vi "MainScreen.vi"() -> ()   [LabVIEW 2020]
uses:
  Source/PN.ctl
  Source/NewPNConfig.ctl
  Source/InputPlanning.ctl
  <vilib>/Utility/miscctls.llb/LVRowAndColumnTypeDef.ctl
  85a98836-3ca8-4481-b4b7-f46a48c72065.vi
  <vilib>/Array/Sort 2D Array - Pop Stack.vi
  <vilib>/Array/Sort 2D Array - Push Stack.vi
  <vilib>/Utility/config.llb/Read Key (String).vi
  <vilib>/Utility/config.llb/Write Key (String).vi
  <vilib>/Utility/file.llb/Read Delimited Spreadsheet (string).vi
  <vilib>/Utility/file.llb/Write Delimited Spreadsheet (string).vi
  <vilib>/regexp/Match Regular Expression.xnode
  <vilib>/Utility/config.llb/NI_LVConfig.lvlib
panel:
  out "error out 4":errorcluster
  out "Version":string
  out "Boolean":bool
  out "ConfigPath":string
  out "Check":dbl
  out "TempFolder":string
  out "SeqPath":string
  in  "stop":bool
  out "TestStandPath":string
  in  "Tab1":T1(tab)
  in  "CurrentStatus":string[][](table)
  in  "Remove Button":bool
  out "CurrentQueue":string[][](table)
  in  "SAVE_Plan":bool
  in  "RESET_Queue":bool
  in  "InputParameter":T2
  in  "EditFlow":bool
  in  "SAVEConfig":bool
  in  "ConfigLoad":T3 {"Screw 8" items=["0", "1", "2", "3", "4", "5", "6", "7", "8", "9", "10"]; "Screw 7" items=["0", "1", "2", "3", "4", "5", "6", "7", "8", "9", "10"]; "Screw 6" items=["0", "1", "2", "3", "4", "5", "6", "7", "8", "9", "10"]; "Screw 5" items=["0", "1", "2", "3", "4", "5", "6", "7", "8", "9", "10"]; "Screw 4" items=["0", "1", "2", "3", "4", "5", "6", "7", "8", "9", "10"]; "Screw 3" items=["0", "1", "2", "3", "4", "5", "6", "7", "8", "9", "10"]; "Screw 2" items=["0", "1", "2", "3", "4", "5", "6", "7", "8", "9", "10"]; "M6_Camera" items=["0", "1", "2", "3", "4", "5", "6", "7", "8", "9", "10", "11", "12", "13", "14", "15", "16", "17", "18", "19", "20", "21", "22", "23", "24", "25", "26", "27", "28", "29", "30"]; "L/R" items=["NA", "RHD-VAC", "RHD-HVAC", "LHD-VAC", "LHD-HVAC"]}
  out "Layout":string[](array[string])=["VALEO PN", "LEFT/RIGHT", "SCREW"]
  in  "CurrentSeq":T4
  in  "String 2":string="EDIT PN"
  in  "CreateNewPN":bool
  in  "String":string="NEW PN"
  in  "New PN":string
  in  "Note":string[](array[string])
  in  "Control":bool[][](array[boolean])
  out "Input":bool[][](array[boolean])
  out "MAP":string[][](array[string])
  out "Slave Status":u32[](array[colorbox])
  in  "ManualMachine":bool
  in  "Select PN to send to Machine":T4
  in  "Select Machine for Manual Test":T4
  in  "StartRun":bool
  # "s1"
  # "s2"
  # "s3"
  # "s4"
  # "s5"
  # "s6"
  # "s7"
  # "s8"
  # "s9"
  # "s10"
  # "s11"
  # "s12"
  # "s13"
  # "s14"
  # "s15"
  # "s16"
  # "s17"
  # "s18"
  # "s19"
  # "s20"
  # "s21"
  # "s22"
  # "s23"
  # "s24"
  # "s25"
  # "s26"
  # "s27"
  # "s28"
  # "s29"
  # "s30"
  # "s31"
  # "P2"
  # "P1"
  # "P3"
  # "P0"
  # "P0"
  # "P1"
  # "P2"
  # "P3"
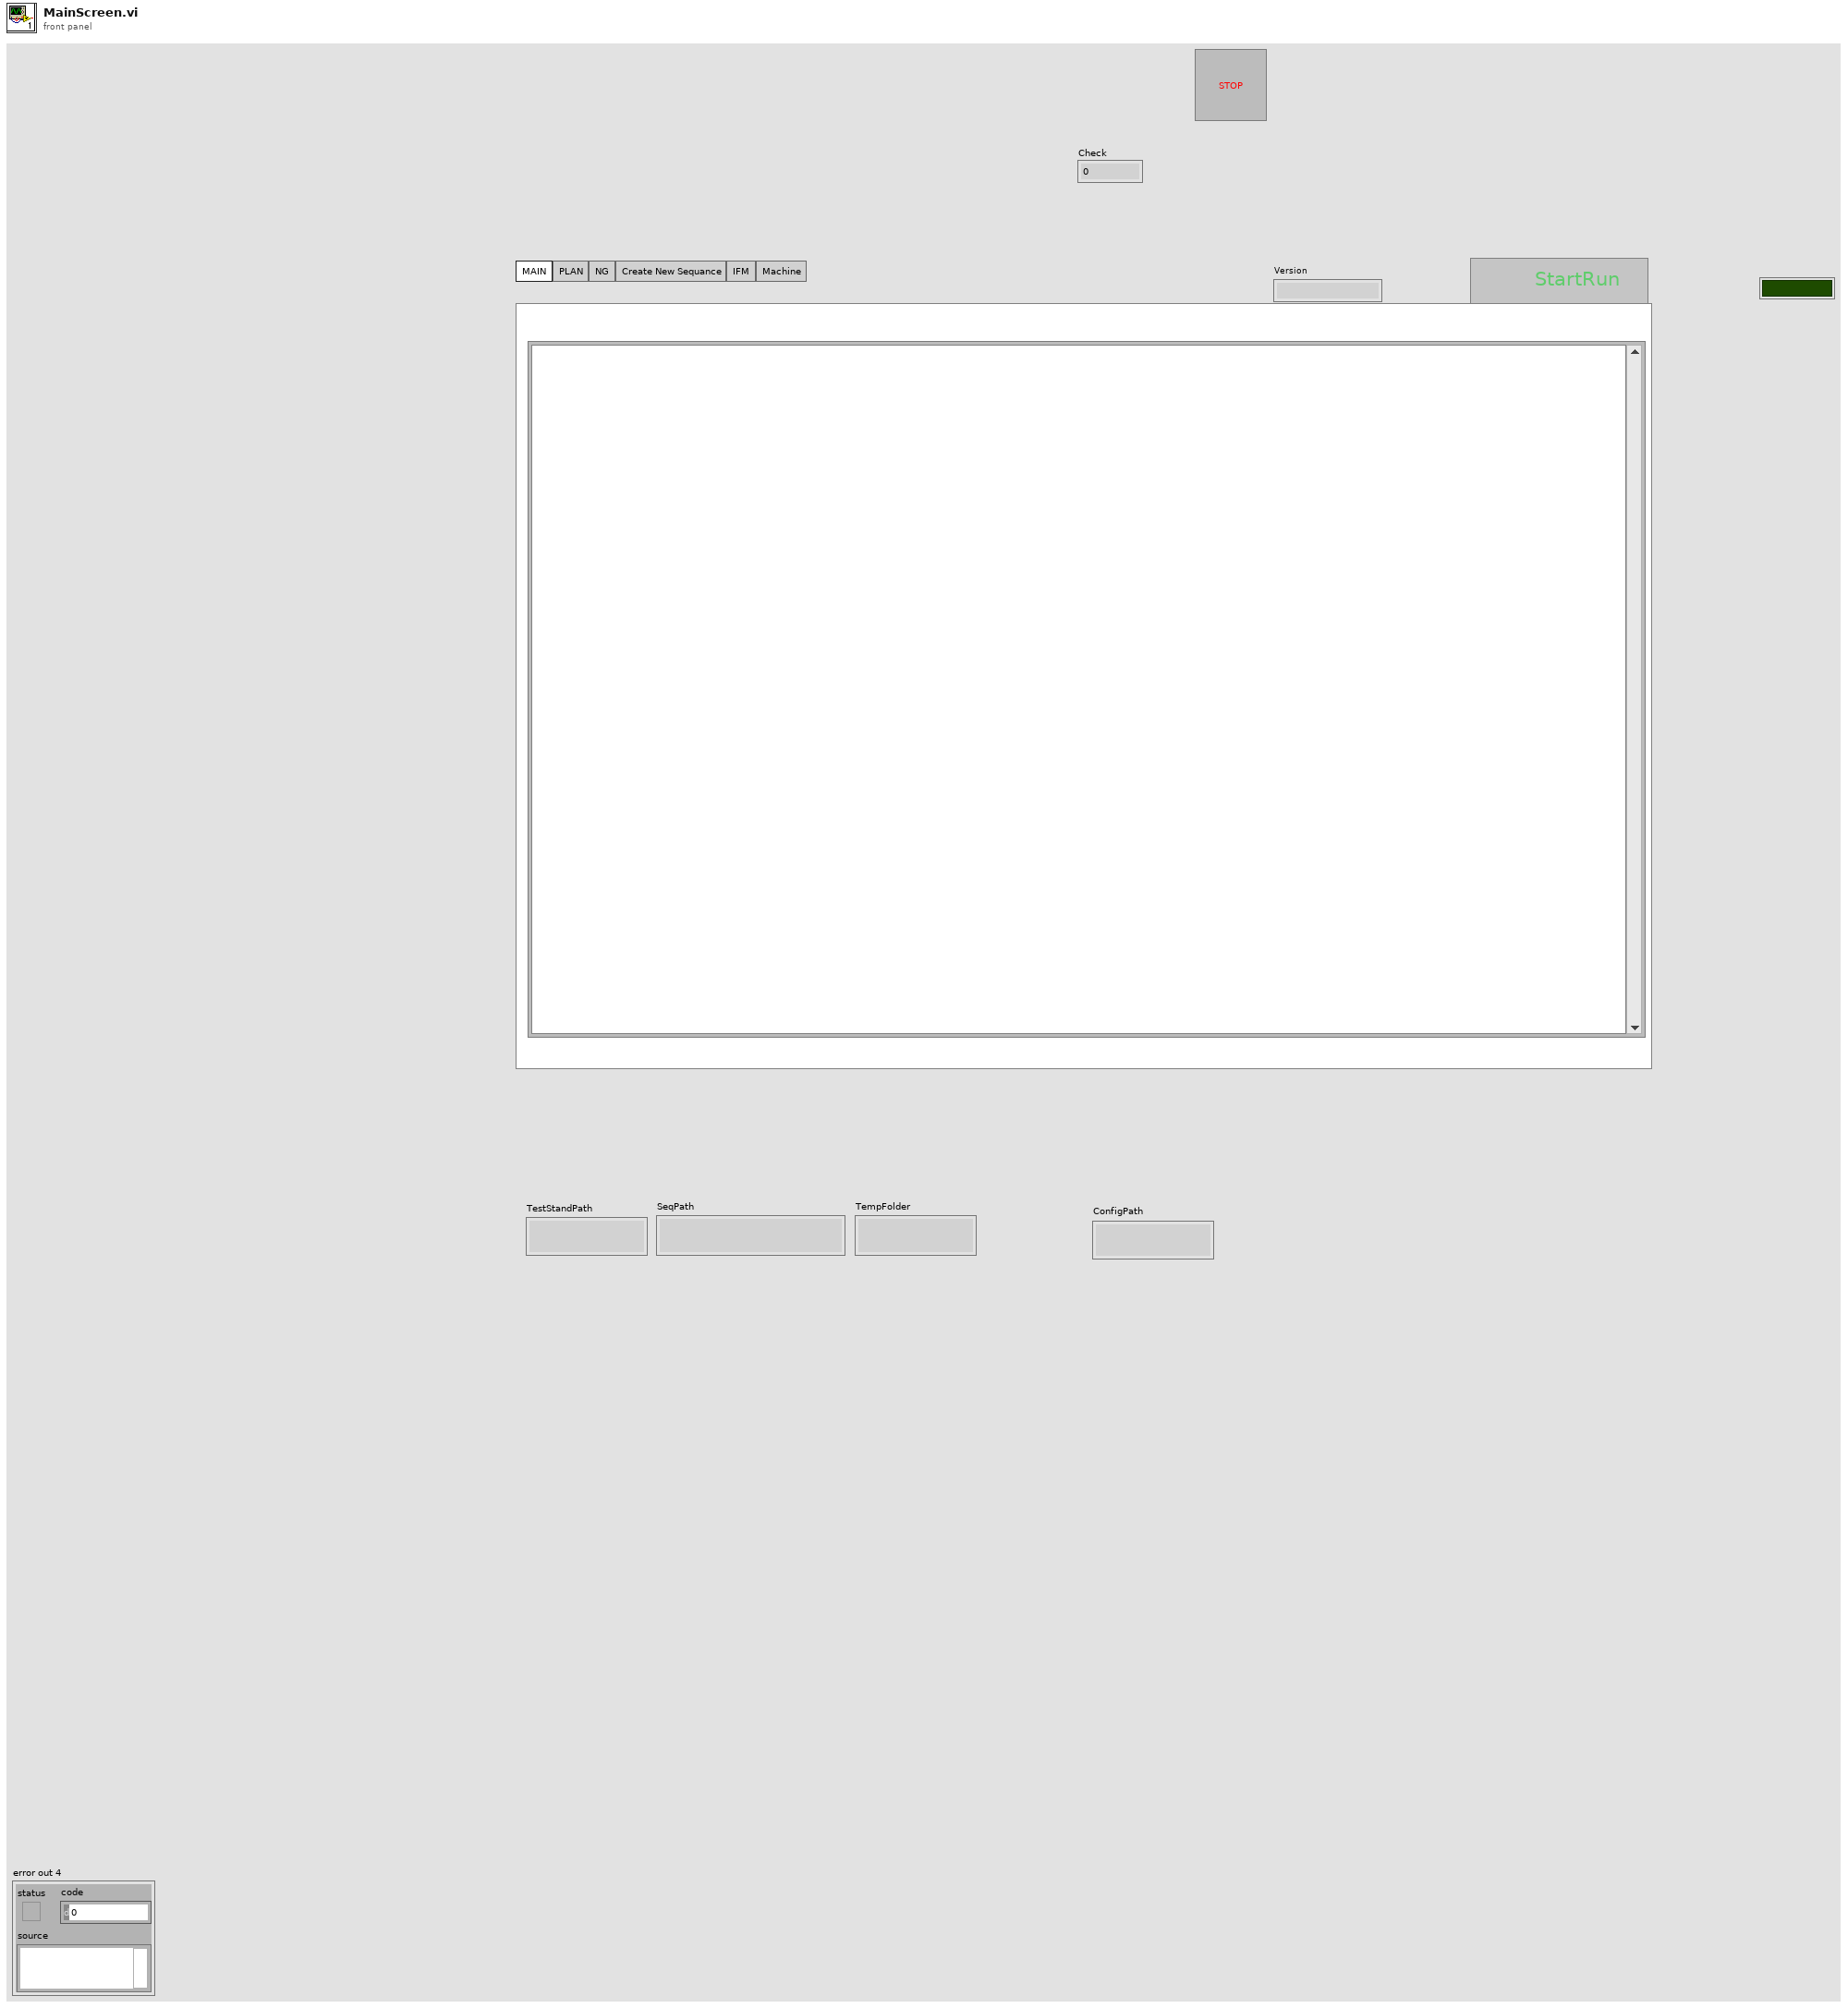
[diagram p1: front panel]
types:
  T1 = enum32{"MAIN", "PLAN", "NG", "Create New Sequance", "IFM", "Machine"}
  T2 = typedef "InputPlanning.ctl" = cluster{"Count":i16, "PN":string}[]
  T3 = typedef "NewPNConfig.ctl" = cluster{"L/R":u8, "PN":string, "M6_Camera":u16, "Screw 2":u16, "Screw 3":u16, "Screw 4":u16, "Screw 5":u16, "Screw 6":u16, "Screw 7":u16, "Screw 8":u16}
  T4 = typedef "PN.ctl" = string
  T5 = enum8{"Enabled", "Disabled", "Disabled and Grayed Out"}
  T6 = enum32{"MAIN", "PLAN", "NG", "Create New Sequance"}
  T7 = typedef "NI_LVConfig.lvlib/Config Data RefNum.ctl" = refnum<k1>
  T8 = typedef "LVRowAndColumnTypeDef.ctl" = cluster{"Row":i32, "Column":i32}
  T9 = cluster{"FileVersion":string, "FileMajorPart":i32, "FileMinorPart":i32, "FileBuildPart":i32, "FilePrivatePart":i32, "Language":string, "LegalCopyright":string, "FileDescription":string, "CompanyName":string, "ProductName":string, "InternalName":string}
  T10 = cluster{"Read Access":enum8{"Allowed", "Required", "None"}, "Write Access":enum8{"Allowed", "Required", "None"}}
  T11 = enum16{"open", "replace", "create", "open or create", "replace or create", "replace or create with confirmation"}
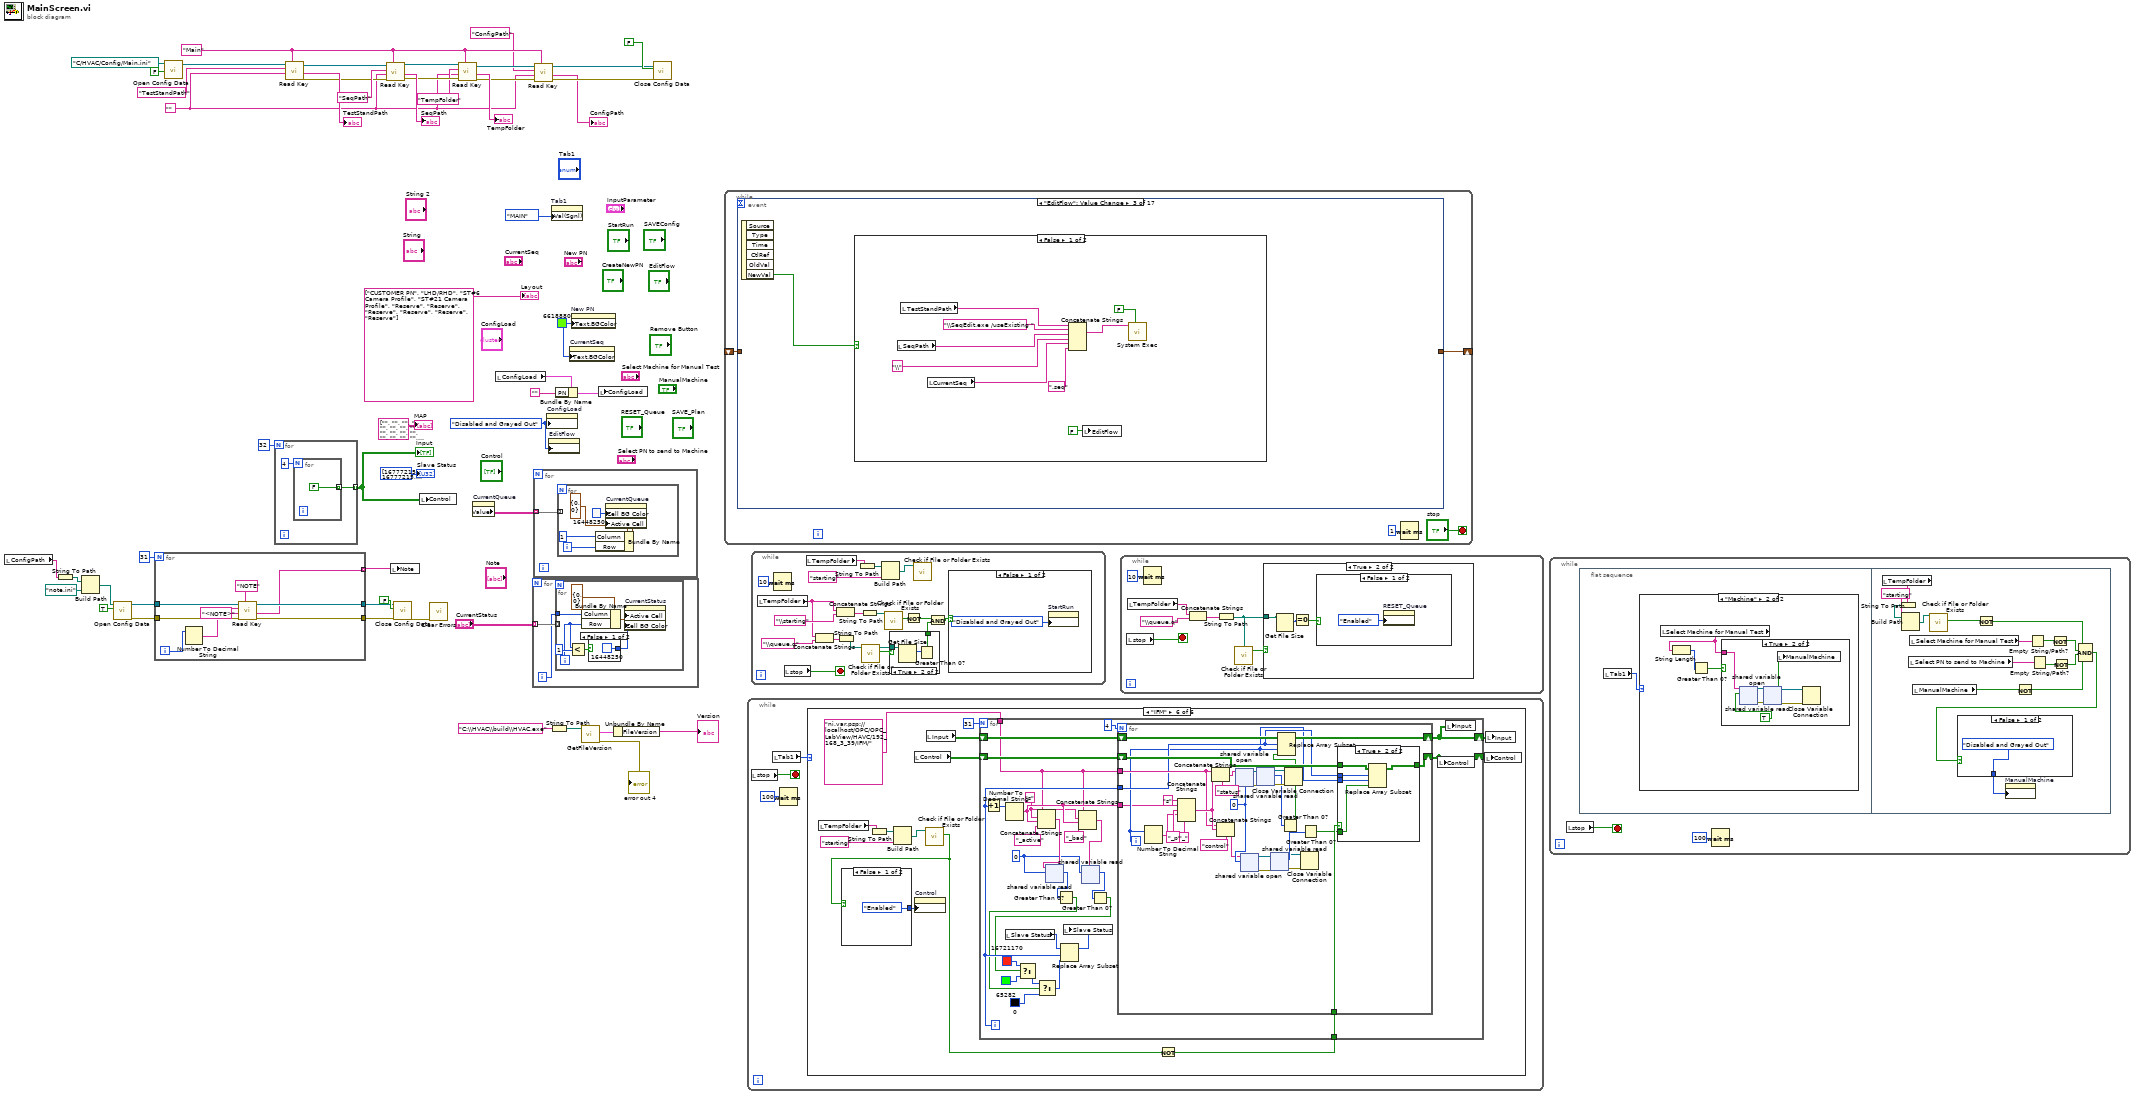
[diagram p0: block diagram]
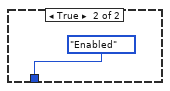
[diagram p4: hidden frame]
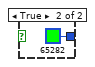
[diagram p5: hidden frame]
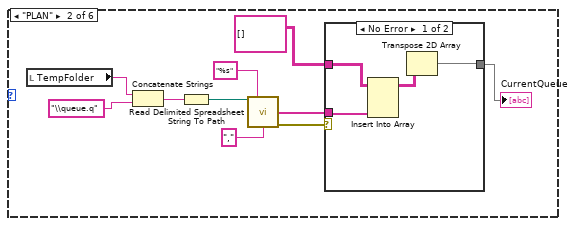
[diagram p7: hidden frame]
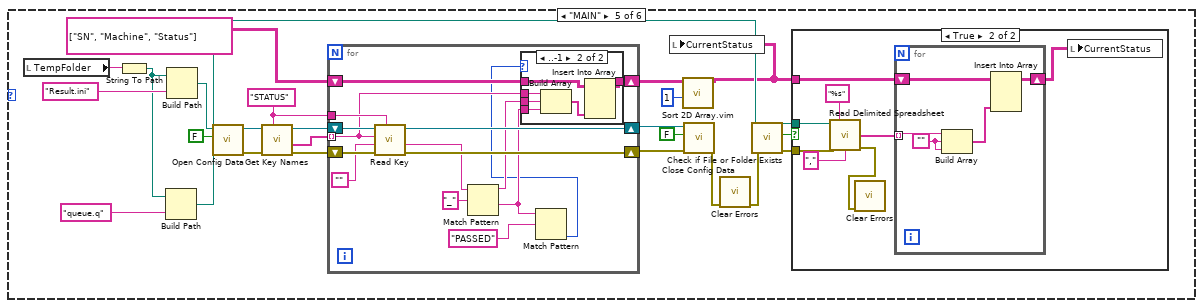
[diagram p11: hidden frame]
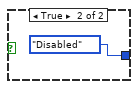
[diagram p14: hidden frame]
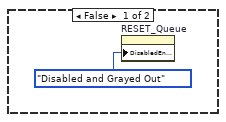
[diagram p16: hidden frame]
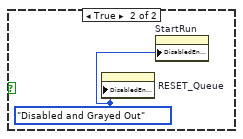
[diagram p17: hidden frame]
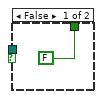
[diagram p18: hidden frame]
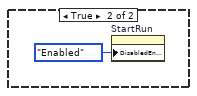
[diagram p19: hidden frame]
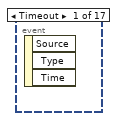
[diagram p20: hidden frame]
diagram:
  w26 = T5."Disabled and Grayed Out" ("Disabled")
  w39 = u32 6618880 ("Text.Text Colors:BG Color")
  w35 = ""
  w34 = "Main" ("section")
  n1 = local read "ConfigPath"() -> (w11:string)
  n2 = String To Path(string=w11) -> (path=w12:path)
  n3 = Build Path(base path=w12, name or relative path=path "note.ini") -> (appended path=w9:path)
  n4 = call <vilib>:"Open Config Data.vi"("create file if necessary (T)"=TRUE, "configuration file path"=w9) -> ("error out"=w3:errorcluster, "refnum"=w6:T7)  [unwired: 7 in, 1 out]
  n5 = for {
    N: 31 -> [_]
    tunnel: w6 -> [w60]
    tunnel: [w59] -> w5
    tunnel: [w58] -> w4
    tunnel: w3 -> [w57]
    tunnel: [w54] -> w2 mode=indexing
    i -> [w56]
    n6 = Number To Decimal String(number=w56) -> (decimal integer string=w55:string)  [unwired: 1 in]
    n7 = call-poly <vilib>:"Read Key.vi"("section"="NOTE", "error in (no error)"=w57, "default value"="<NOTE>", "key"=w55, "refnum"=w60) -> ("error out"=w58:errorcluster, "value"=w54:string, "refnum out"=w59:T7)  [unwired: 3 in, 1 out]
  }
  n8 = call <vilib>:"Open Config Data.vi"("create file if necessary (T)"=FALSE, "configuration file path"=path "C:/HVAC/Config/Main.ini") -> ("refnum"=w51:T7)  [unwired: 7 in, 2 out]
  n9 = for {
    N: 32 -> [_]
    tunnel: [w63] -> w21 mode=indexing
    n10 = for {
      N: 4 -> [_]
      tunnel: [FALSE] -> w63 mode=indexing
    }
  }
  "Input" <- w21
  n11 = call-poly <vilib>:"Read Key.vi"("section"=w34, "default value"=w35, "key"="TestStandPath", "refnum"=w51) -> ("error out"=w45:errorcluster, "value"=→"TestStandPath":string, "refnum out"=w46:T7)  [unwired: 4 in, 1 out]
  n12 = call-poly <vilib>:"Read Key.vi"("section"=w34, "error in (no error)"=w45, "default value"=w35, "key"="SeqPath", "refnum"=w46) -> ("error out"=w43:errorcluster, "value"=→"SeqPath":string, "refnum out"=w42:T7)  [unwired: 3 in, 1 out]
  n13 = local write "Note"(w2) -> ()
  n14 = call <vilib>:"Close Config Data.vi"("error in (no error)"=w4, "write file if changed (T)"=FALSE, "refnum"=w5) -> ("error out"=w1:errorcluster)  [unwired: 7 in, 1 out]
  n15 = local write "Control"(w21) -> ()
  n16 = call <vilib>:"Clear Errors.vi"("error in (no error)"=w1) -> ()  [unwired: 5 in, 2 out]
  n17 = call-poly <vilib>:"Read Key.vi"("section"=w34, "error in (no error)"=w43, "default value"=w35, "key"="TempFolder", "refnum"=w42) -> ("error out"=w37:errorcluster, "value"=→"TempFolder":string, "refnum out"=w36:T7)  [unwired: 3 in, 1 out]
  n18 = property on="CurrentQueue" class="Tbl (strict)"() -> ("Value"=w24:string[][])  [unwired: 2 in, 2 out]
  n19 = local read "ConfigLoad"() -> (w29:T3)
  n20 = for {
    tunnel: "CurrentStatus" -> [w67] mode=indexing
    i -> [w66]
    n21 = for {
      tunnel: w67 -> [_] mode=indexing
      tunnel: w66 -> [w69]
      i -> [w68]
      n22 = Less?(x=w68, y=1) -> (x < y?=w71:bool)
      n23 = Bundle By Name(cluster=T8 {"Row"=0, "Column"=0} ("Active Cell:Active Cell"), "Column"=w69, "Row"=w68) -> (w72:T8)
      n24 = case shown="False" w71 {
        tunnel: [u32 16448250 ("Active Cell:Cell Background Color") u32 65282 ("Active Cell:Cell Background Color")] -> w74
        frame False {
        }
        frame True {
        }
      }
      n25 = property on="CurrentStatus" class="Tbl (strict)"("Active Cell"=w72, "Cell BG Color"=w74) -> ()  [unwired: 2 in, 2 out]
    }
  }
  n26 = for {
    tunnel: w24 -> [w77] mode=indexing
    n27 = for {
      tunnel: w77 -> [_] mode=indexing
      i -> [w78]
      n28 = Bundle By Name(cluster=T8 {"Row"=0, "Column"=0} ("Active Cell:Active Cell"), "Column"=1, "Row"=w78) -> (w80:T8)
      n29 = property on="CurrentQueue" class="Tbl (strict)"("Cell BG Color"=u32 16448250 ("Active Cell:Cell Background Color"), "Active Cell"=w80) -> ()  [unwired: 2 in, 2 out]
    }
  }
  n30 = call-poly <vilib>:"Read Key.vi"("section"=w34, "error in (no error)"=w37, "default value"=w35, "key"="ConfigPath", "refnum"=w36) -> ("error out"=w32:errorcluster, "value"=→"ConfigPath":string, "refnum out"=w33:T7)  [unwired: 3 in, 1 out]
  n31 = property on="ConfigLoad" class="Clust (strict)"("DisabledEnum"=w26) -> ()  [unwired: 2 in, 2 out]
  n32 = property on="EditFlow" class="Bool (strict)"("DisabledEnum"=w26) -> ()  [unwired: 2 in, 2 out]
  n33 = String To Path(string="C:\\HVAC\\build\\HVAC.exe") -> (path=w16:path)
  n34 = property on="Tab1" class="TabCtl (strict)"("Val(Sgnl)"=T6."MAIN" ("Tab1")) -> ()  [unwired: 2 in, 2 out]
  n35 = Bundle By Name(cluster=w29, "PN"="") -> (w28:T3)
  n36 = property on="CurrentSeq" class="CmbBox (strict)"("Text.BGColor"=w39) -> ()  [unwired: 2 in, 2 out]
  n37 = property on="New PN" class="Str"("Text.BGColor"=w39) -> ()  [unwired: 2 in, 2 out]
  n38 = call "GetFileVersion.vi"("Exe Path"=w16) -> ("error out"=→"error out 4":errorcluster, "File Info Out"=w17:T9)  [unwired: 8 in, 1 out]
  n39 = local write "ConfigLoad"(w28) -> ()
  n40 = Unbundle By Name(w17) -> ("FileVersion"=→"Version":string)
  n41 = call <vilib>:"Close Config Data.vi"("error in (no error)"=w32, "write file if changed (T)"=FALSE, "refnum"=w33) -> ()  [unwired: 7 in, 2 out]
  n42 = while {
    shift-right: [w84] -> _
    shift-left: _ -> [w83]
    stop <- "stop" stop-if-true
    n43 = event shown="[2] \"EditFlow\": Value Change" {
      selector: _ -> [_ _ _ _ _ _ _ _ _ _ _ _ _ _ _ _ _]
      dyn-events: _ -> [_ _ _ _ _ _ _ _ _ _ _ _ _ _ _ _ _]
      timeout: _ -> [_ _ _ _ _ _ _ _ _ _ _ _ _ _ _ _ _]
      tunnel: [_ _ _ _ _ _ _ _ _ _ w453 _ _ _ _ _ _] -> w84
      tunnel: w83 -> [_ _ _ _ _ _ _ _ _ _ w443 _ _ _ _ _ _]
      event Timeout {
        n44 = event-data() -> ()  [unwired: 1 in, 3 out]
      }
      event "StartRun": Value Change {
        n45 = event-data() -> ("NewVal"=w87:bool)  [unwired: 1 in, 5 out]
        n46 = case shown="False" w87 {
          frame False {
            n47 = local read "SeqPath"() -> (w93:string)
            n48 = local read "TestStandPath"() -> (w91:string)
            n49 = local write "StartRun"(FALSE ("StartRun")) -> ()
            n50 = Concatenate Strings(w91, "\\SeqEdit.exe /useExisting -run MainSequence " ("string"), w93, "\\Main.seq") -> (w90:string)
            n51 = call <vilib>:"System Exec.vi"("wait until completion? (T)"=FALSE, "command line"=w90) -> ()  [unwired: 6 in, 4 out]
          }
          frame True {
          }
        }
      }
      event "EditFlow": Value Change {
        n52 = event-data() -> ("NewVal"=w95:bool)  [unwired: 1 in, 5 out]
        n53 = case shown="False" w95 {
          frame False {
            n54 = local read "SeqPath"() -> (w103:string)
            n55 = local read "TestStandPath"() -> (w101:string)
            n56 = local read "CurrentSeq"() -> (w97:T4)
            n57 = Concatenate Strings(w101, "\\SeqEdit.exe /useExisting " ("string"), w103, "\\", w97, ".seq" ("string")) -> (w100:string)
            n58 = local write "EditFlow"(FALSE ("EditFlow")) -> ()
            n59 = call <vilib>:"System Exec.vi"("wait until completion? (T)"=FALSE, "command line"=w100) -> ()  [unwired: 6 in, 4 out]
          }
          frame True {
          }
        }
      }
      event "Tab1": Value Change {
        n60 = event-data() -> ("NewVal"=w105:T1)  [unwired: 1 in, 5 out]
        "Check" <- w105
        n61 = case shown="\"IFM\"" w105 {
          frame "MAIN", Default {
          }
          frame "Machine" {
            w110 = "ni.var.psp://localhost/OPC/OPC_LabView/HAVC/192_168_3_39/PLC/"
            n62 = Search Variable Container(10:"^(.*)Start" ("regular expression"), 11:w110) -> (2:w112:refnum<k21>[])  [unwired: 4 in, 2 out]
            n63 = local read "SeqPath"() -> (w109:string)
            n64 = for {
              tunnel: w112 -> [w119] mode=indexing
              tunnel: [w120] -> w111 mode=indexing
              tunnel: w110 -> [w118]
              n65 = Match Pattern(string=w119, regular expression=w118) -> (after substring=w117:string)  [unwired: 1 in, 3 out]
              n66 = Match Pattern(string=w117, regular expression="Start") -> (before substring=w115:string)  [unwired: 1 in, 3 out]
              n67 = case shown="\"STROBO\"" w115 {
                selector: w115 -> [w122 _ _]
                tunnel: [w122 "Vision" "EOL"] -> w114
                frame Default {
                }
                frame "STROBO" {
                }
                frame "STEOL" {
                }
              }
              n68 = Bundle By Name(cluster=cluster{"String":string, "Value":string} {"String"="", "Value"=""} ("element"), "String"=w114, "Value"=w119) -> (w120:cluster{"String":string, "Value":string})
            }
            n69 = call "ListSEQFile.vi"("Path"=w109) -> ("SEQ Path"=w108:string[])  [unwired: 10 in]
            n70 = property on="Select PN to send to Machine" class="CmbBox (strict)"("Strings[]"=w108, "Value"="") -> ()  [unwired: 2 in, 2 out]
            n71 = property on="Select Machine to Manual Test" class="CmbBox (strict)"("Strings And Values[]"=w111, "Value"="") -> ()  [unwired: 2 in, 2 out]
          }
          frame "NG" {
          }
          frame "Create New Sequance" {
            w125 = T5."Disabled and Grayed Out" ("Disabled")
            n72 = local read "SeqPath"() -> (w129:string)
            n73 = call "ListSEQFile.vi"("Path"=w129) -> ("SEQ Path"=w128:string[])  [unwired: 10 in]
            n74 = local write "New PN"("INPUT NEW PN/SCAN." ("Value (Signaling)")) -> ()
            n75 = property on="CurrentSeq" class="CmbBox (strict)"("Strings[]"=w128, "Value"="NA" ("Value (Signaling)")) -> ()  [unwired: 2 in, 2 out]
            n76 = property on="EditFlow" class="Bool (strict)"("DisabledEnum"=w125) -> ()  [unwired: 2 in, 2 out]
            n77 = property on="SAVEConfig" class="Bool (strict)"("DisabledEnum"=w125) -> ()  [unwired: 2 in, 2 out]
          }
          frame "PLAN" {
            n78 = local read "InputParameter"() -> (w132:T2)
            n79 = local read "SeqPath"() -> (w134:string)
            n80 = call "ListSEQFile.vi"("Path"=w134) -> ("SEQ Path"=w130:string[])  [unwired: 10 in]
            n81 = property on="PN" class="CmbBox"("Strings[]"=w130) -> ()  [unwired: 2 in, 2 out]
            n82 = for {
              N: 13 -> [_]
              tunnel: w130 -> [w141]
              shift-right: [w139] -> w131
              shift-left: w132 -> [w138]
              w137 = 0 ("index")
              n83 = Index Array(array=w141, index=w137) -> (element=w140:string)
              n84 = Index Array(array=w138, index=w137) -> (element=w136:cluster{"Count":i16, "PN":string})
              n85 = Bundle By Name(cluster=w136, "PN"=w140, "Count"=w137) -> (w135:cluster{"Count":i16, "PN":string})
              n86 = Insert Into Array(array=w138, new element=w135) -> (w139:T2)  [unwired: 1 in]
            }
            n87 = local write "InputParameter"(w131) -> ()
          }
          frame "IFM" {
            n88 = local read "MAP"() -> (w143:string[][])
            n89 = Open/Create/Replace File(file path (use dialog)=path "C:/HVAC/Config/Main.ini", access (0:read/write)=enum16{"read/write", "read-only", "write-only"}."read-only") -> (refnum out=w150:refnum<file>, error out=w151:errorcluster)  [unwired: 4 in, 1 out]
            n90 = Read from Text File(file (use dialog)=w150, error in=w151) -> (refnum out=w148:refnum<file>, text=w145:string, error out=w149:errorcluster)  [unwired: 2 in, 1 out]
            n91 = for {
              N: 31 -> [_]
              tunnel: w148 -> [w160]
              shift-right: [w162] -> w147
              shift-left: w149 -> [w163]
              tunnel: [w161] -> w146
              tunnel: w145 -> [w159]
              shift-right: [w155] -> w142
              shift-left: w143 -> [w156]
              i -> [w154]
              n92 = Increment(x=w154) -> (x+1=w157:i32)
              n93 = Number To Decimal String(number=w154) -> ()  [unwired: 1 in, 1 out]
              n94 = for {
                N: 4 -> [_]
                shift-right: [w183] -> w162
                shift-left: w163 -> [w183]
                tunnel: [w182] -> w161
                tunnel: w160 -> [w182]
                tunnel: w159 -> [w175]
                tunnel: w157 -> [w181]
                tunnel: w154 -> [w169]
                shift-right: [w171] -> w155
                shift-left: w156 -> [w170]
                i -> [w168]
                n95 = Number To Decimal String(number=w181) -> (decimal integer string=w179:string)  [unwired: 1 in]
                n96 = Number To Decimal String(number=w168) -> (decimal integer string=w177:string)  [unwired: 1 in]
                n97 = Concatenate Strings("^(.*)=\"s" ("string"), w179, "_p" ("string"), w177) -> (w176:string)
                n98 = xnode "Match Regular Expression"("input string"=w175, "regular expression"=w176, "multiline? (F)"=TRUE) -> ("whole match"=w172:string)  [unwired: 3 in, 4 out]
                n99 = Match Pattern(string=w172, regular expression="=") -> (before substring=w167:string)  [unwired: 1 in, 3 out]
                n100 = Search and Replace String(input string=w167, search string="SCREW_", replace string="SC_" ("replace string (\"\")")) -> (result string=w166:string)  [unwired: 5 in, 3 out]
                n101 = Replace Array Subset(array=w170, new element=w166, index (row)=w169, index (col)=w168) -> (w171:string[][])
              }
            }
            n102 = local write "MAP"(w142) -> ()
            n103 = Close File(refnum=w146, error in=w147) -> ()  [unwired: 2 out]
          }
        }
      }
      event "Note": Value Change {
        n104 = event-data() -> ("OldVal"=w299:string[], "NewVal"=w298:string[])  [unwired: 1 in, 4 out]
        n105 = for {
          tunnel: w299 -> [w303] mode=indexing
          tunnel: w298 -> [w301] mode=indexing
          i -> [w300]
          n106 = Not Equal?(x=w303, y=w301) -> (x != y?=w302:bool)
          n107 = case shown="True" w302 {
            tunnel: w301 -> [_ w310]
            tunnel: w300 -> [_ w308]
            frame False {
            }
            frame True {
              n108 = Number To Decimal String(number=w308) -> (decimal integer string=w307:string)  [unwired: 1 in]
              n109 = local read "ConfigPath"() -> (w316:string)
              n110 = String To Path(string=w316) -> (path=w317:path)
              n111 = Build Path(base path=w317, name or relative path=path "note.ini") -> (appended path=w314:path)
              n112 = call <vilib>:"Open Config Data.vi"("create file if necessary (T)"=TRUE, "configuration file path"=w314) -> ("error out"=w311:errorcluster, "refnum"=w312:T7)  [unwired: 7 in, 1 out]
              n113 = call-poly <vilib>:"Write Key.vi"("section"="NOTE", "error in (no error)"=w311, "value"=w310, "key"=w307, "refnum"=w312) -> ("error out"=w306:errorcluster, "refnum out"=w305:T7)  [unwired: 4 in, 1 out]
              n114 = call <vilib>:"Close Config Data.vi"("error in (no error)"=w306, "write file if changed (T)"=TRUE, "refnum"=w305) -> ()  [unwired: 7 in, 2 out]
            }
          }
        }
      }
      event "ManualMachine": Value Change {
        n115 = event-data() -> ("NewVal"=w318:bool)  [unwired: 1 in, 5 out]
        n116 = case shown="True" w318 {
          frame False {
          }
          frame True {
            n117 = local read "Select PN to send to Machine"() -> (w326:T4)
            n118 = local read "Select Machine for Manual Test"() -> (w323:T4)
            n119 = Match Pattern(string=w323, regular expression="PLC/ST") -> (after substring=w321:T4)  [unwired: 1 in, 3 out]
            n120 = Match Pattern(string=w321, regular expression="Start") -> (before substring=w319:T4)  [unwired: 1 in, 3 out]
            n121 = Concatenate Strings(w326, "_99" ("string")) -> (w324:string)
            n122 = call "MachineControl.vi"("Station"=w319, "SN"=w324) -> ()  [unwired: 6 in, 4 out]
          }
        }
      }
      event "CreateNewPN": Value Change {
        n123 = event-data() -> ("NewVal"=w327:bool)  [unwired: 1 in, 5 out]
        n124 = local read "SeqPath"() -> (w334:string)
        n125 = local read "New PN"() -> (w328:string)
        n126 = Concatenate Strings(w334, "\\" ("string"), w328, ".seq" ("string")) -> (w330:string)
        n127 = String To Path(string=w330) -> (path=w331:path)
        n128 = call <vilib>:"Check if File or Folder Exists.vi"("path"=w331) -> ("file or folder exists?"=w329:bool)  [unwired: 8 in, 2 out]
        n129 = case shown="False" w327 {
          tunnel: w329 -> [w336 _]
          tunnel: w328 -> [w335 _]
          frame False {
            n130 = case shown="False" w336 {
              tunnel: w335 -> [_ w360]
              frame False {
                n131 = local read "ConfigPath"() -> (w337:string)
                n132 = local read "New PN"() -> (w339:string)
                n133 = call "NewPNConfig.vi"("Path"=w337, "Config for PN"=w339) -> ("OK"=w338:bool)  [unwired: 7 in, 2 out]
                n134 = case shown="True" w338 {
                  tunnel: w337 -> [_ w342]
                  frame False {
                    n135 = local write "CreateNewPN"(FALSE ("CreateNewPN")) -> ()
                  }
                  frame True {
                    n136 = local read "New PN"() -> (w343:string)
                    n137 = local read "SeqPath"() -> (w352:string)
                    n138 = local write "CreateNewPN"(FALSE ("CreateNewPN")) -> ()
                    n139 = Concatenate Strings(w352, "\\FullRun.seq" ("element")) -> (w348:string)
                    n140 = Concatenate Strings(w352, "\\" ("string"), w343, ".seq" ("string")) -> (w349:string)
                    n141 = String To Path(string=w348) -> (path=w347:path)
                    n142 = String To Path(string=w349) -> (path=w346:path)
                    n143 = Copy(9:TRUE ("overwrite (F)"), 10:w346, 11:w347) -> (0:w344:errorcluster)  [unwired: 2 in, 2 out]
                    n144 = case shown="No Error" w344 {
                      tunnel: w343 -> [w356 _]
                      tunnel: w342 -> [w355 _]
                      frame No Error {
                        n145 = local read "SeqPath"() -> (w358:string)
                        n146 = call "ListSEQFile.vi"("Path"=w358) -> ("SEQ Path"=w357:string[])  [unwired: 10 in]
                        n147 = property on="CurrentSeq" class="CmbBox (strict)"("Strings[]"=w357, "Value"=w356) -> ()  [unwired: 2 in, 2 out]
                        n148 = call "LoadConfig.vi"("Path"=w355, "PN"=w356) -> ("Cluster"=w354:T3)  [unwired: 9 in]
                        n149 = local write "ConfigLoad"(w354) -> ()
                      }
                      frame Error {
                      }
                    }
                  }
                }
              }
              frame True {
                n150 = flat-sequence {
                  tunnel: w360 -> [w362]
                  tunnel: [w362] -> w359
                  tunnel: w359 -> [w365]
                  frame #0 {
                    n151 = local write "CreateNewPN"(FALSE ("CreateNewPN")) -> ()
                    n152 = One Button Dialog(message="PN exists, Go to EDIT instead. ") -> ()  [unwired: 1 in, 1 out]
                  }
                  frame #1 {
                    w364 = T5."Enabled" ("Disabled")
                    n153 = local read "ConfigPath"() -> (w368:string)
                    n154 = local write "CurrentSeq"(w365) -> ()
                    n155 = property on="ConfigLoad" class="Clust (strict)"("DisabledEnum"=T5."Enabled" ("Disabled")) -> ()  [unwired: 2 in, 2 out]
                    n156 = property on="CreateNewPN" class="Bool (strict)"("DisabledEnum"=T5."Disabled and Grayed Out" ("Disabled")) -> ()  [unwired: 2 in, 2 out]
                    n157 = property on="SAVEConfig" class="Bool (strict)"("DisabledEnum"=w364) -> ()  [unwired: 2 in, 2 out]
                    n158 = property on="EditFlow" class="Bool (strict)"("DisabledEnum"=w364) -> ()  [unwired: 2 in, 2 out]
                    n159 = call "LoadConfig.vi"("Path"=w368, "PN"=w365) -> ("Cluster"=w367:T3)  [unwired: 9 in]
                    n160 = local write "ConfigLoad"(w367) -> ()
                  }
                }
              }
            }
          }
          frame True {
          }
        }
      }
      event "Control": Value Change {
        n161 = event-data() -> ("OldVal"=w375:bool[][], "NewVal"=w376:bool[][])  [unwired: 1 in, 4 out]
        n162 = local read "TempFolder"() -> (w373:string)
        n163 = String To Path(string=w373) -> (path=w372:path)
        n164 = Build Path(base path=w372, name or relative path="starting") -> (appended path=w371:path)
        n165 = call <vilib>:"Check if File or Folder Exists.vi"("path"=w371) -> ("file or folder exists?"=w370:bool)  [unwired: 8 in, 2 out]
        n166 = case shown="False" w370 {
          tunnel: w376 -> [w378 _]
          tunnel: w375 -> [w377 _]
          frame False {
            n167 = for {
              tunnel: w378 -> [w382] mode=indexing
              tunnel: w377 -> [w381] mode=indexing
              i -> [w380]
              n168 = Increment(x=w380) -> (x+1=w379:i32)
              n169 = for {
                tunnel: w382 -> [w383] mode=indexing
                tunnel: w381 -> [w389] mode=indexing
                tunnel: w379 -> [w384]
                i -> [w385]
                n170 = Number To Decimal String(number=w384) -> (decimal integer string=w386:string)  [unwired: 1 in]
                n171 = Number To Decimal String(number=w385) -> (decimal integer string=w387:string)  [unwired: 1 in]
                n172 = Equal?(x=w389, y=w383) -> (x = y?=w388:bool)
                n173 = case shown="False" w388 {
                  tunnel: w387 -> [w401 _]
                  tunnel: w386 -> [w403 _]
                  tunnel: w383 -> [w397 _]
                  frame False {
                    n174 = Boolean To (0,1)(Boolean=w397) -> (0, 1=w390:i16)
                    n175 = Concatenate Strings("s", w403, "_p" ("string"), w401, "_control" ("string")) -> (w399:string)
                    n176 = Concatenate Strings("ni.var.psp://localhost/OPC/OPC_LabView/HAVC/192_168_3_39/IFM/", w399) -> (w392:string)
                    n177 = shared-variable-open(w392, w390, T10 {"Read Access"=enum."Allowed", "Write Access"=enum."Allowed"} ("access")) -> (w393:refnum<k21>, w394:errorcluster)  [unwired: 1 in]
                    n178 = while {
                      tunnel: w390 -> [w410]
                      tunnel: [w409] -> w396
                      tunnel: [w408] -> w395
                      tunnel: w394 -> [w407]
                      tunnel: w393 -> [w406]
                      stop <- w411 stop-if-true
                      n179 = shared-variable-write(w406, w407, w410) -> (w405:refnum<k21>, w414:errorcluster)
                      n180 = call "Time Delay"("error in (no error)"=w414) -> ("error out"=w413:errorcluster)  [unwired: 10 in]
                      n181 = shared-variable-read(w405, w413) -> (w408:refnum<k21>, w409:errorcluster, w412:i16)  [unwired: 1 out]
                      n182 = Equal?(x=w412, y=w410) -> (x = y?=w411:bool)
                    }
                    n183 = Close Variable Connection(8:w396, 11:w395) -> ()  [unwired: 1 out]
                  }
                  frame True {
                  }
                }
              }
            }
          }
          frame True {
          }
        }
      }
      event Value Change {
        n184 = event-data() -> ("NewVal"=w415:T4)  [unwired: 1 in, 5 out]
        n185 = Not Equal?(x=w415, y="NA") -> (x != y?=w417:bool)
        n186 = String Length(string=w415) -> (length=w419:i32)
        n187 = Greater Than 0?(x=w419) -> (x > 0?=w418:bool)
        n188 = And(x=w417, y=w418) -> (x .and. y?=w416:bool)
        n189 = case shown="True" w416 {
          tunnel: w415 -> [_ w429]
          frame False {
            w421 = T5."Disabled and Grayed Out" ("Disabled")
            n190 = local read "ConfigLoad"() -> (w423:T3)
            n191 = Bundle By Name(cluster=w423, "PN"="") -> (w424:T3)
            n192 = property on="SAVEConfig" class="Bool (strict)"("DisabledEnum"=w421) -> ()  [unwired: 2 in, 2 out]
            n193 = property on="EditFlow" class="Bool (strict)"("DisabledEnum"=w421) -> ()  [unwired: 2 in, 2 out]
            n194 = property on="ConfigLoad" class="Clust (strict)"("DisabledEnum"=T5."Disabled and Grayed Out" ("Disabled")) -> ()  [unwired: 2 in, 2 out]
            n195 = local write "ConfigLoad"(w424) -> ()
          }
          frame True {
            w426 = T5."Enabled" ("Disabled")
            n196 = local read "ConfigPath"() -> (w428:string)
            n197 = property on="ConfigLoad" class="Clust (strict)"("DisabledEnum"=T5."Enabled" ("Disabled")) -> ()  [unwired: 2 in, 2 out]
            n198 = call "LoadConfig.vi"("Path"=w428, "PN"=w429) -> ("Cluster"=w430:T3)  [unwired: 9 in]
            n199 = property on="EditFlow" class="Bool (strict)"("DisabledEnum"=w426) -> ()  [unwired: 2 in, 2 out]
            n200 = property on="SAVEConfig" class="Bool (strict)"("DisabledEnum"=w426) -> ()  [unwired: 2 in, 2 out]
            n201 = local write "ConfigLoad"(w430) -> ()
          }
        }
      }
      event "SAVEConfig": Value Change {
        n202 = event-data() -> ("NewVal"=w431:bool)  [unwired: 1 in, 5 out]
        n203 = local read "ConfigLoad"() -> (w435:T3)
        n204 = Unbundle By Name(w435) -> ("PN"=w434:string)
        n205 = String Length(string=w434) -> (length=w433:i32)
        n206 = Greater Than 0?(x=w433) -> (x > 0?=w432:bool)
        n207 = case shown="False" w431 {
          tunnel: w432 -> [w436 _]
          frame False {
            n208 = case shown="True" w436 {
              frame False {
                n209 = local write "SAVEConfig"(FALSE ("SAVEConfig")) -> ()
                n210 = One Button Dialog(message="Please make sure the CUSTOMER PN cannot Blank.") -> ()  [unwired: 1 in, 1 out]
              }
              frame True {
                n211 = local read "CurrentSeq"() -> (w441:T4)
                n212 = local read "ConfigPath"() -> (w442:string)
                n213 = local read "ConfigLoad"() -> (w440:T3)
                n214 = local write "SAVEConfig"(FALSE ("SAVEConfig")) -> ()
                n215 = call "SaveConfig.vi"("Cluster"=w440, "PN"=w441, "Path"=w442) -> ()  [unwired: 8 in, 1 out]
              }
            }
          }
          frame True {
          }
        }
      }
      event "CurrentQueue": Mouse Down {
        n216 = event-data() -> ()  [unwired: 1 in, 8 out]
        n217 = property on="CurrentQueue" class="Tbl (strict)"() -> ("Number of Columns"=w450:u32)  [unwired: 2 in, 2 out]
        n218 = property on="CurrentQueue" class="Tbl (strict)"() -> ("Selection Start"=w453:T8, "Value"=w448:string[][])  [unwired: 2 in, 2 out]
        n219 = Unbundle By Name(w443) -> ("Row"=w451:i32)  [unwired: 1 out]
        n220 = Unbundle By Name(w453) -> ("Row"=w447:i32, "Column"=w446:i32)
        n221 = Index Array(array=w448, index (row)=w447, index (col)=w446) -> (element=w445:string)
        n222 = String Length(string=w445) -> (length=w449:i32)
        n223 = Greater Than 0?(x=w449) -> (x > 0?=w444:bool)
        n224 = case shown="True" w444 {
          tunnel: w447 -> [_ w456]
          tunnel: w453 -> [_ w455]
          tunnel: w450 -> [_ w454]
          frame False {
          }
          frame True {
            n225 = for {
              N: w454 -> [_]
              tunnel: u32 6618880 -> [w458]
              tunnel: w455 -> [w462]
              tunnel: w456 -> [w461]
              i -> [w460]
              n226 = Bundle(cluster=w462, "Row"=w461, "Column"=w460) -> (w459:T8)
              n227 = property on="CurrentQueue" class="Tbl (strict)"("Active Cell"=w459, "Cell BG Color"=w458) -> ()  [unwired: 2 in, 2 out]
            }
          }
        }
        n228 = for {
          N: w450 -> [_]
          tunnel: u32 16448250 -> [w464]
          tunnel: w443 -> [w467]
          tunnel: w451 -> [w466]
          i -> [w465]
          n229 = Bundle(cluster=w467, "Row"=w466, "Column"=w465) -> (w463:T8)
          n230 = property on="CurrentQueue" class="Tbl (strict)"("Active Cell"=w463, "Cell BG Color"=w464) -> ()  [unwired: 2 in, 2 out]
        }
      }
      event "Remove Button": Value Change {
        n231 = event-data() -> ("NewVal"=w468:bool)  [unwired: 1 in, 5 out]
        n232 = case shown="False" w468 {
          frame False {
            w475 = "," ("delimiter (\\t)")
            w473 = "%s" ("format (%s)")
            n233 = property on="CurrentQueue" class="Tbl (strict)"() -> ("Active Cell"=w471:T8)  [unwired: 2 in, 2 out]
            n234 = local read "TempFolder"() -> (w482:string)
            n235 = String To Path(string=w482) -> (path=w481:path)
            n236 = Unbundle By Name(w471) -> ("Row"=w483:i32)
            n237 = Build Path(base path=w481, name or relative path="queue.q") -> (appended path=w479:path)
            n238 = call-poly <vilib>:"Read Delimited Spreadsheet.vi"("file path (dialog if empty)"=w479, "format (%s)"=w473, "delimiter (\\t)"=w475) -> ("new file path (Not A Path if cancelled)"=w476:path, "first row"=w478:string[])  [unwired: 7 in, 4 out]
            n239 = Delete From Array(array=w478, length=1, index=w483) -> (array with subset deleted=w474:string[])  [unwired: 1 out]
            n240 = local write "Remove Button"(FALSE ("Remove Button")) -> ()
            n241 = call-poly <vilib>:"Write Delimited Spreadsheet.vi"("file path (dialog if empty)"=w476, "format (%s)"=w473, "1D data"=w474, "append to file? (new file:F)"=FALSE, "delimiter (\\t)"=w475) -> ("error out"=w470:errorcluster)  [unwired: 9 in, 1 out]
            n242 = property on="CurrentQueue" class="Tbl (strict)"(error in=w470, "Cell BG Color"=u32 16448250 ("Active Cell:Cell Background Color")) -> ()  [unwired: 1 in, 2 out]
          }
          frame True {
          }
        }
      }
      event "New PN": Mouse Enter {
        n243 = event-data() -> ()  [unwired: 1 in, 4 out]
        n244 = local read "New PN"() -> (w485:string)
        n245 = Equal?(x="INPUT NEW PN/SCAN." ("Value (Signaling)"), y=w485) -> (x = y?=w486:bool)
        n246 = Select(t="", s=w486, f=w485) -> (s? t:f=w487:string)
        n247 = property on="New PN" class="Str"("Val(Sgnl)"=w487, "Text.TextColor"=u32 0 ("Text.Text Colors:Text Color")) -> ()  [unwired: 2 in, 2 out]
      }
      event "New PN": Value Change {
        n248 = event-data() -> ()  [unwired: 1 in, 6 out]
        n249 = local read "New PN"() -> (w495:string)
        n250 = String Length(string=w495) -> (length=w494:i32)
        n251 = Equal?(x="INPUT NEW PN/SCAN." ("Value (Signaling)"), y=w495) -> (x = y?=w497:bool)
        n252 = Greater Than 0?(x=w494) -> (x > 0?=w493:bool)
        n253 = Not(x=w497) -> (.not. x?=w496:bool)
        n254 = And(x=w496, y=w493) -> (x .and. y?=w492:bool)
        n255 = case shown="True" w492 {
          tunnel: [T5."Disabled and Grayed Out" ("Disabled") T5."Enabled" ("Disabled")] -> w491
          frame False {
          }
          frame True {
          }
        }
        n256 = property on="CreateNewPN" class="Bool (strict)"("DisabledEnum"=w491) -> ()  [unwired: 2 in, 2 out]
      }
      event "New PN": Mouse Leave {
        n257 = event-data() -> ()  [unwired: 1 in, 4 out]
        n258 = local read "New PN"() -> (w502:string)
        n259 = String Length(string=w502) -> (length=w501:i32)
        n260 = case shown="..0" w501 {
          frame Default {
          }
          frame ..0 {
            n261 = property on="New PN" class="Str"("Val(Sgnl)"="INPUT NEW PN/SCAN." ("Value (Signaling)"), "Text.TextColor"=u32 10122868 ("Text.Text Colors:Text Color")) -> ()  [unwired: 2 in, 2 out]
          }
        }
      }
      event "RESET_Queue": Value Change {
        n262 = event-data() -> ("NewVal"=w505:bool)  [unwired: 1 in, 5 out]
        n263 = case shown="False" w505 {
          frame False {
            n264 = local write "RESET_Queue"(FALSE ("RESET_Queue")) -> ()
            n265 = local read "TempFolder"() -> (w509:string)
            n266 = Concatenate Strings(w509, "\\starting") -> (w508:string)
            n267 = Concatenate Strings(w509, "\\queue.q") -> (w516:string)
            n268 = String To Path(string=w508) -> (path=w507:path)
            n269 = String To Path(string=w516) -> (path=w515:path)
            n270 = Delete(path (use dialog)=w507) -> (error out=w506:errorcluster)  [unwired: 4 in, 2 out]
            n271 = call-poly <vilib>:"Write Delimited Spreadsheet.vi"("file path (dialog if empty)"=w515, "format (%s)"="%s" ("format (%.3f)"), "1D data"=string[] [], "append to file? (new file:F)"=FALSE, "delimiter (\\t)"="," ("delimiter (\\t)")) -> ()  [unwired: 9 in, 2 out]
            n272 = case shown="No Error" w506 {
              frame No Error {
              }
              frame Error {
              }
            }
          }
          frame True {
          }
        }
      }
      event "SAVE_Plan": Value Change {
        n273 = event-data() -> ("NewVal"=w519:bool)  [unwired: 1 in, 5 out]
        n274 = case shown="False" w519 {
          frame False {
            w528 = "%s" ("format (%.3f)")
            n275 = local read "TempFolder"() -> (w535:string)
            n276 = local read "InputParameter"() -> (w530:T2)
            n277 = local write "SAVE_Plan"(FALSE ("SAVE_Plan")) -> ()
            n278 = Concatenate Strings(w535, "\\queue.q") -> (w534:string)
            n279 = String To Path(string=w534) -> (path=w524:path)
            n280 = Open/Create/Replace File(file path (use dialog)=w524, operation (0:open)=T11."open or create") -> (refnum out=w521:refnum<file>, error out=w522:errorcluster)  [unwired: 4 in, 1 out]
            n281 = Close File(refnum=w521, error in=w522) -> (path=w520:path)  [unwired: 1 out]
            n282 = call-poly <vilib>:"Read Delimited Spreadsheet.vi"("file path (dialog if empty)"=w520, "format (%s)"=w528, "delimiter (\\t)"="," ("delimiter (\\t)")) -> ("first row"=w526:string[])  [unwired: 7 in, 5 out]
            n283 = for {
              tunnel: w530 -> [w540] mode=indexing
              shift-right: [w545] -> w529
              shift-left: w526 -> [w546]
              tunnel: [w537] -> w525 mode=indexing
              n284 = Unbundle By Name(w540) -> ("Count"=w541:i16, "PN"=w548:string)
              n285 = Bundle By Name(cluster=w540, "PN"="NA", "Count"=i16 0) -> (w537:cluster{"Count":i16, "PN":string})
              n286 = Not Equal?(x=w548, y="NA") -> (x != y?=w543:bool)
              n287 = Greater Than 0?(x=w541) -> (x > 0?=w544:bool)
              n288 = And(x=w543, y=w544) -> (x .and. y?=w542:bool)
              n289 = case shown="True" w542 {
                tunnel: w541 -> [_ w553]
                tunnel: w548 -> [_ w552]
                tunnel: w546 -> [w549 w551]
                tunnel: [w549 w550] -> w545
                frame False {
                }
                frame True {
                  n290 = for {
                    N: w553 -> [_]
                    tunnel: w552 -> [w563]
                    shift-right: [w557] -> w550
                    shift-left: w551 -> [w554]
                    n291 = Array Size(array=w554) -> (size(s)=w561:i32)
                    n292 = Concatenate Strings(w563, "_" ("regular expression")) -> (w562:string)
                    n293 = while {
                      tunnel: w554 -> [w572] mode=indexing
                      tunnel: [w572] -> _
                      tunnel: w562 -> [w571]
                      tunnel: w561 -> [w569]
                      tunnel: [w566] -> w556 mode=indexing
                      i -> [w570]
                      stop <- w568 stop-if-true
                      n294 = Greater Or Equal?(x=w570, y=w569) -> (x >= y?=w568:bool)
                      n295 = xnode "Match Regular Expression"("input string"=w572, "regular expression"=w571) -> ("after match"=w567:string)  [unwired: 4 in, 4 out]
                      n296 = Decimal String To Number(string=w567) -> (number=w566:i32)  [unwired: 2 in, 1 out]
                    }
                    n297 = Array Max & Min(array=w556) -> (max value=w555:i32)  [unwired: 3 out]
                    n298 = Increment(x=w555) -> (x+1=w560:i32)
                    n299 = Number To Decimal String(number=w560) -> (decimal integer string=w559:string)  [unwired: 1 in]
                    n300 = Concatenate Strings(w563, "_" ("string"), w559) -> (w558:string)
                    n301 = Insert Into Array(array=w554, new element=w558) -> (w557:string[])  [unwired: 1 in]
                  }
                }
              }
            }
            n302 = local write "InputParameter"(w525) -> ()
            n303 = call-poly <vilib>:"Write Delimited Spreadsheet.vi"("file path (dialog if empty)"=w524, "format (%s)"=w528, "1D data"=w529, "append to file? (new file:F)"=FALSE, "delimiter (\\t)"="," ("delimiter (\\t)")) -> ()  [unwired: 9 in, 2 out]
          }
          frame True {
          }
        }
      }
    }
    n304 = Wait (ms)(milliseconds to wait=u32 1) -> ()  [unwired: 1 out]
  }
  n305 = while {
    stop <- w688 stop-if-true
    n306 = local read "stop"() -> (w688:bool)
    n307 = local read "Tab1"() -> (w687:T1)
    n308 = Wait (ms)(milliseconds to wait=u32 100) -> ()  [unwired: 1 out]
    n309 = case shown="\"IFM\"" w687 {
      frame Default {
      }
      frame "PLAN" {
        n310 = local read "TempFolder"() -> (w698:string)
        n311 = Concatenate Strings(w698, "\\queue.q") -> (w699:string)
        n312 = String To Path(string=w699) -> (path=w696:path)
        n313 = call-poly <vilib>:"Read Delimited Spreadsheet.vi"("file path (dialog if empty)"=w696, "format (%s)"="%s", "delimiter (\\t)"="," ("delimiter (\\t)")) -> ("first row"=w693:string[], "error out"=w694:errorcluster)  [unwired: 7 in, 4 out]
        n314 = case shown="No Error" w694 {
          tunnel: w693 -> [w702 _]
          tunnel: string[][] [] ("CurrentQueue") -> [w703 w704]
          tunnel: [w700 w704] -> w690
          frame No Error {
            n315 = Insert Into Array(array=w703, new element=w702) -> (w701:string[][])  [unwired: 2 in]
            n316 = Transpose 2D Array(2D array=w701) -> (transposed array=w700:string[][])
          }
          frame Error {
          }
        }
        "CurrentQueue" <- w690
      }
      frame "NG" {
      }
      frame "Create New Sequance" {
      }
      frame "MAIN" {
        w720 = "STATUS" ("section")
        n317 = local read "TempFolder"() -> (w729:string)
        n318 = String To Path(string=w729) -> (path=w715:path)
        n319 = Build Path(base path=w715, name or relative path="queue.q") -> (appended path=w713:path)
        n320 = Build Path(base path=w715, name or relative path="Result.ini" ("time format string (%c)")) -> (appended path=w727:path)
        n321 = call <vilib>:"Open Config Data.vi"("create file if necessary (T)"=FALSE, "configuration file path"=w727) -> ("error out"=w725:errorcluster, "refnum"=w724:T7)  [unwired: 7 in, 1 out]
        n322 = call <vilib>:"Get Key Names.vi"("section"=w720, "error in (no error)"=w725, "refnum"=w724) -> ("error out"=w722:errorcluster, "key names"=w721:string[], "refnum out"=w723:T7)  [unwired: 5 in, 1 out]
        n323 = for {
          shift-right: [w753] -> w718
          shift-left: w722 -> [w757]
          shift-right: [w752] -> w717
          shift-left: w723 -> [w756]
          tunnel: w721 -> [w751] mode=indexing
          tunnel: w720 -> [w755]
          shift-right: [w747] -> w707
          shift-left: string[][] [["SN", "Machine", "Status"]] -> [w746]
          n324 = call-poly <vilib>:"Read Key.vi"("section"=w755, "error in (no error)"=w757, "default value"="", "key"=w751, "refnum"=w756) -> ("error out"=w753:errorcluster, "value"=w750:string, "refnum out"=w752:T7)  [unwired: 3 in, 1 out]
          n325 = Match Pattern(string=w750, regular expression="_") -> (before substring=w748:string, after substring=w745:string)  [unwired: 1 in, 2 out]
          n326 = Match Pattern(string=w745, regular expression="PASSED") -> (offset past match=w743:i32)  [unwired: 1 in, 3 out]
          n327 = case shown="..-1" w743 {
            tunnel: w751 -> [_ w764]
            tunnel: w748 -> [_ w763]
            tunnel: [w758 w762] -> w747
            tunnel: w746 -> [w758 w761]
            tunnel: w745 -> [_ w759]
            frame 0.., Default {
            }
            frame ..-1 {
              n328 = Build Array(w764, w763, w759) -> (w760:string[])
              n329 = Insert Into Array(array=w761, new element=w760) -> (w762:string[][])  [unwired: 2 in]
            }
          }
        }
        n330 = call "Sort 2D Array.vim"("index"=1, "2D array"=w707) -> ("sorted 2D array"=w706:string[][])  [unwired: 8 in, 1 out]
        n331 = local write "CurrentStatus"(w706) -> ()
        n332 = call <vilib>:"Close Config Data.vi"("error in (no error)"=w718, "write file if changed (T)"=FALSE, "refnum"=w717) -> ("error out"=w709:errorcluster)  [unwired: 7 in, 1 out]
        n333 = call <vilib>:"Clear Errors.vi"("error in (no error)"=w709) -> ("error out"=w708:errorcluster)  [unwired: 5 in, 1 out]
        n334 = call <vilib>:"Check if File or Folder Exists.vi"("error in (no error)"=w708, "path"=w713) -> ("error out"=w710:errorcluster, "file or folder exists?"=w711:bool, "dup path"=w712:path)  [unwired: 7 in]
        n335 = case shown="True" w711 {
          tunnel: w712 -> [_ w735]
          tunnel: w710 -> [_ w734]
          tunnel: w706 -> [_ w732]
          frame False {
          }
          frame True {
            n336 = call-poly <vilib>:"Read Delimited Spreadsheet.vi"("file path (dialog if empty)"=w735, "format (%s)"="%s" ("format (%.3f)"), "error in (no error)"=w734, "delimiter (\\t)"="," ("delimiter (\\t)")) -> ("first row"=w733:string[], "error out"=w730:errorcluster)  [unwired: 6 in, 4 out]
            n337 = call <vilib>:"Clear Errors.vi"("error in (no error)"=w730) -> ()  [unwired: 5 in, 2 out]
            n338 = for {
              tunnel: w733 -> [w742] mode=indexing
              shift-right: [w738] -> w731
              shift-left: w732 -> [w739]
              w741 = ""
              n339 = Build Array(w742, w741, w741) -> (w740:string[])
              n340 = Insert Into Array(array=w739, new element=w740) -> (w738:string[][])  [unwired: 2 in]
            }
            n341 = local write "CurrentStatus"(w731) -> ()
          }
        }
      }
      frame "IFM" {
        n342 = local read "TempFolder"() -> (w776:string)
        n343 = String To Path(string=w776) -> (path=w775:path)
        n344 = Build Path(base path=w775, name or relative path="starting") -> (appended path=w774:path)
        n345 = local read "Control"() -> (w772:bool[][])
        n346 = call <vilib>:"Check if File or Folder Exists.vi"("path"=w774) -> ("file or folder exists?"=w766:bool)  [unwired: 8 in, 2 out]
        n347 = case shown="False" w766 {
          tunnel: [T5."Enabled" ("Disabled") T5."Disabled" ("Disabled")] -> w767
          frame False {
          }
          frame True {
          }
        }
        n348 = property on="Control" class="Arr (strict)"("DisabledEnum"=w767) -> ()  [unwired: 2 in, 2 out]
        n349 = local read "Input"() -> (w771:bool[][])
        n350 = Not(x=w766) -> (.not. x?=w765:bool)
        n351 = for {
          N: 31 -> [_]
          shift-right: [w803] -> w770
          shift-left: w771 -> [w805]
          shift-right: [w802] -> w769
          shift-left: w772 -> [w804]
          tunnel: "ni.var.psp://localhost/OPC/OPC_LabView/HAVC/192_168_3_39/IFM/" -> [w780]
          tunnel: w765 -> [w801]
          i -> [w790]
          w793 = 0
          w798 = "s" ("string")
          n352 = Increment(x=w790) -> (x+1=w800:i32)
          n353 = Number To Decimal String(number=w800) -> (decimal integer string=w799:string)  [unwired: 1 in]
          n354 = local read "Slave Status"() -> (w792:u32[])
          n355 = Concatenate Strings(w780, w798, w799, "_active" ("string")) -> (w795:string)
          n356 = shared-variable-read(w795, w793) -> (w787:i32)  [unwired: 1 in, 3 out]
          n357 = Greater Than 0?(x=w787) -> (x > 0?=w786:bool)
          n358 = Concatenate Strings(w780, w798, w799, "_bad" ("string")) -> (w794:string)
          n359 = shared-variable-read(w794, w793) -> (w785:i32)  [unwired: 1 in, 3 out]
          n360 = Greater Than 0?(x=w785) -> (x > 0?=w784:bool)
          n361 = Select(t=u32 16721170 ("BG Color"), s=w784, f=u32 65282 ("BG Color")) -> (s? t:f=w789:u32)
          n362 = Select(t=w789, s=w786, f=u32 0 ("BG Color")) -> (s? t:f=w788:u32)
          n363 = Replace Array Subset(array=w792, new element=w788, index=w790) -> (w791:u32[])
          n364 = local write "Slave Status"(w791) -> ()
          n365 = for {
            N: 4 -> [_]
            tunnel: w790 -> [w821]
            shift-right: [w828] -> w803
            shift-left: w805 -> [w830]
            shift-right: [w825] -> w802
            shift-left: w804 -> [w826]
            tunnel: w780 -> [w829]
            tunnel: w801 -> [w827]
            tunnel: w799 -> [w819]
            i -> [w820]
            w808 = i8 0
            n366 = Number To Decimal String(number=w820) -> (decimal integer string=w835:string)  [unwired: 1 in]
            n367 = Concatenate Strings("s" ("string"), w819, "_p" ("string"), w835, "_" ("string")) -> (w833:string)
            n368 = Concatenate Strings(w829, w833, "status" ("string")) -> (w813:string)
            n369 = Concatenate Strings(w829, w833, "control" ("string")) -> (w807:string)
            n370 = shared-variable-open(w813, w808) -> (w814:refnum<k21>, w815:errorcluster)  [unwired: 2 in]
            n371 = shared-variable-open(w807, w808) -> (w812:refnum<k21>, w811:errorcluster)  [unwired: 2 in]
            n372 = shared-variable-read(w814, w815) -> (w817:refnum<k21>, w818:errorcluster, w816:i8)  [unwired: 1 out]
            n373 = shared-variable-read(w812, w811) -> (w809:refnum<k21>, w810:errorcluster, w824:i8)  [unwired: 1 out]
            n374 = Greater Than 0?(x=w816) -> (x > 0?=w823:bool)
            n375 = Replace Array Subset(array=w830, new element=w823, index (row)=w821, index (col)=w820) -> (w828:bool[][])
            n376 = Close Variable Connection(8:w818, 11:w817) -> ()  [unwired: 1 out]
            n377 = Close Variable Connection(8:w810, 11:w809) -> ()  [unwired: 1 out]
            n378 = Greater Than 0?(x=w824) -> (x > 0?=w822:bool)
            n379 = case shown="True" w827 {
              tunnel: w826 -> [w838 w843]
              tunnel: [w838 w839] -> w825
              tunnel: w822 -> [_ w840]
              tunnel: w821 -> [_ w842]
              tunnel: w820 -> [_ w841]
              frame False {
              }
              frame True {
                n380 = Replace Array Subset(array=w843, new element=w840, index (row)=w842, index (col)=w841) -> (w839:bool[][])
              }
            }
          }
          n381 = local write "Control"(w802) -> ()
          n382 = local write "Input"(w803) -> ()
        }
        n383 = local write "Control"(w769) -> ()
        n384 = local write "Input"(w770) -> ()
      }
    }
  }
  n385 = while {
    stop <- w862 stop-if-true
    n386 = local read "TempFolder"() -> (w857:string)
    n387 = Wait (ms)(milliseconds to wait=u32 10) -> ()  [unwired: 1 out]
    n388 = local read "stop"() -> (w862:bool)
    n389 = local read "TempFolder"() -> (w845:string)
    n390 = Concatenate Strings(w857, "\\queue.q") -> (w855:string)
    n391 = Concatenate Strings(w857, "\\starting") -> (w859:string)
    n392 = String To Path(string=w855) -> (path=w854:path)
    n393 = String To Path(string=w845) -> (path=w846:path)
    n394 = String To Path(string=w859) -> (path=w858:path)
    n395 = call <vilib>:"Check if File or Folder Exists.vi"("path"=w854) -> ("file or folder exists?"=w853:bool, "dup path"=w852:path)  [unwired: 8 in, 1 out]
    n396 = Build Path(base path=w846, name or relative path="starting") -> (appended path=w847:path)
    n397 = call <vilib>:"Check if File or Folder Exists.vi"("path"=w858) -> ("file or folder exists?"=w851:bool)  [unwired: 8 in, 2 out]
    n398 = case shown="True" w853 {
      tunnel: w852 -> [_ w866]
      tunnel: [FALSE w864] -> w848
      frame False {
      }
      frame True {
        n399 = Get File Size(file=w866) -> (size (in bytes)=w865:i64)  [unwired: 1 in, 2 out]
        n400 = Greater Than 0?(x=w865) -> (x > 0?=w864:bool)
      }
    }
    n401 = Not(x=w851) -> (.not. x?=w850:bool)
    n402 = call <vilib>:"Check if File or Folder Exists.vi"("path"=w847) -> ()  [unwired: 8 in, 3 out]
    n403 = And(x=w850, y=w848) -> (x .and. y?=w849:bool)
    n404 = case shown="False" w849 {
      frame False {
        n405 = property on="StartRun" class="Bool (strict)"("DisabledEnum"=T5."Disabled and Grayed Out" ("Disabled")) -> ()  [unwired: 2 in, 2 out]
      }
      frame True {
        n406 = property on="StartRun" class="Bool (strict)"("DisabledEnum"=T5."Enabled" ("Disabled")) -> ()  [unwired: 2 in, 2 out]
      }
    }
  }
  n407 = while {
    stop <- w875 stop-if-true
    n408 = local read "stop"() -> (w875:bool)
    n409 = local read "TempFolder"() -> (w872:string)
    n410 = Wait (ms)(milliseconds to wait=u32 10) -> ()  [unwired: 1 out]
    n411 = Concatenate Strings(w872, "\\queue.q") -> (w871:string)
    n412 = String To Path(string=w871) -> (path=w869:path)
    n413 = call <vilib>:"Check if File or Folder Exists.vi"("path"=w869) -> ("file or folder exists?"=w870:bool)  [unwired: 8 in, 2 out]
    n414 = case shown="True" w870 {
      tunnel: w869 -> [_ w877]
      frame False {
        n415 = property on="RESET_Queue" class="Bool (strict)"("DisabledEnum"=T5."Disabled and Grayed Out" ("Disabled")) -> ()  [unwired: 2 in, 2 out]
      }
      frame True {
        n416 = Get File Size(file=w877) -> (size (in bytes)=w879:i64)  [unwired: 1 in, 2 out]
        n417 = Equal To 0?(x=w879) -> (x = 0?=w878:bool)
        n418 = case shown="False" w878 {
          frame False {
            n419 = property on="RESET_Queue" class="Bool (strict)"("DisabledEnum"=T5."Enabled" ("Disabled")) -> ()  [unwired: 2 in, 2 out]
          }
          frame True {
            w881 = T5."Disabled and Grayed Out" ("Disabled")
            n420 = property on="RESET_Queue" class="Bool (strict)"("DisabledEnum"=w881) -> ()  [unwired: 2 in, 2 out]
            n421 = property on="StartRun" class="Bool (strict)"("DisabledEnum"=w881) -> ()  [unwired: 2 in, 2 out]
          }
        }
      }
    }
  }
  n422 = while {
    stop <- w883 stop-if-true
    n423 = local read "stop"() -> (w883:bool)
    n424 = flat-sequence {
      frame #0 {
        n425 = local read "Tab1"() -> (w884:T1)
        n426 = case shown="\"Machine\"" w884 {
          frame Default {
          }
          frame "Machine" {
            n427 = local read "Select Machine for Manual Test"() -> (w885:T4)
            n428 = String Length(string=w885) -> (length=w886:i32)
            n429 = Greater Than 0?(x=w886) -> (x > 0?=w887:bool)
            n430 = case shown="True" w887 {
              tunnel: w885 -> [_ w888]
              frame False {
              }
              frame True {
                n431 = shared-variable-open(w888, TRUE) -> (w892:refnum<k21>, w893:errorcluster)  [unwired: 2 in]
                n432 = shared-variable-read(w892, w893) -> (w891:refnum<k21>, w890:errorcluster, w894:bool)  [unwired: 1 out]
                n433 = local write "ManualMachine"(w894) -> ()
                n434 = Close Variable Connection(8:w890, 11:w891) -> ()  [unwired: 1 out]
              }
            }
          }
        }
      }
      frame #1 {
        n435 = local read "TempFolder"() -> (w910:string)
        n436 = String To Path(string=w910) -> (path=w909:path)
        n437 = Build Path(base path=w909, name or relative path="starting") -> (appended path=w907:path)
        n438 = local read "Select PN to send to Machine"() -> (w902:T4)
        n439 = local read "Select Machine for Manual Test"() -> (w901:T4)
        n440 = local read "ManualMachine"() -> (w898:bool)
        n441 = call <vilib>:"Check if File or Folder Exists.vi"("path"=w907) -> ("file or folder exists?"=w896:bool)  [unwired: 8 in, 2 out]
        n442 = Not(x=w896) -> (.not. x?=w895:bool)
        n443 = Not(x=w898) -> (.not. x?=w897:bool)
        n444 = Empty String/Path?(string/path=w901) -> (empty?=w903:bool)
        n445 = Empty String/Path?(string/path=w902) -> (empty?=w904:bool)
        n446 = Not(x=w903) -> (.not. x?=w906:bool)
        n447 = Not(x=w904) -> (.not. x?=w905:bool)
        n448 = Compound Arithmetic op=AND(w895, w906, w905, w897) -> (w899:bool)
        n449 = case shown="False" w899 {
          tunnel: [T5."Disabled and Grayed Out" ("Disabled") T5."Enabled" ("Disabled")] -> w900
          frame False {
          }
          frame True {
          }
        }
        n450 = property on="ManualMachine" class="Bool (strict)"("DisabledEnum"=w900) -> ()  [unwired: 2 in, 2 out]
      }
    }
    n451 = Wait (ms)(milliseconds to wait=u32 100) -> ()  [unwired: 1 out]
  }
  "Layout" <- string[] ["CUSTOMER PN", "LHD/RHD", "ST#6 Camera Profile", "ST#21 Camera Profile", "Reserve", "Reserve", "Reserve", "Reserve", "Reserve", "Reserve"] ("Layout")
  "Slave Status" <- u32[] [16777215, 16777215, 16777215, 16777215, 16777215, 16777215, 16777215, 16777215, 16777215, 16777215, 16777215, 16777215, 16777215, 16777215, 16777215, 16777215, 16777215, 16777215, 16777215, 16777215, 16777215, 16777215, 16777215, 16777215, 16777215, 16777215, 16777215, 16777215, 16777215, 16777215, 16777215, 16777215, 16448250] ("Status")
  "MAP" <- string[][] [["", "", "", "", ""], ["", "", "", "", ""], ["", "", "", "", ""], ["", "", "", "", ""], ["", "", "", "", ""], ["25", "", "", "", ""], ["", "", "", "", ""], ["", "", "", "", ""], ["", "", "", "", ""], ["", "", "", "", ""], ["", "", "", "", ""], ["", "", "", "", ""], ["", "", "", "", ""], ["", "", "", "", ""], ["", "", "", "", ""], ["", "", "", "", ""], ["", "", "", "", ""], ["", "", "", "", ""], ["", "", "", "", ""], ["20", "", "", "", ""], ["", "", "", "", ""], ["", "", "", "", ""], ["", "", "", "", ""], ["", "", "", "", ""], ["", "", "", "", ""], ["", "", "", "", ""], ["", "", "", "", ""], ["", "", "", "", ""], ["", "", "", "", ""], ["", "", "", "", ""], ["", "", "", "", ""], ["", "", "", "", ""], ["", "", "", "", " "]] ("MAP")
